vi "Write Data.vi"(8 "error in (no error)":errorcluster, 10 "Data":sgl, 11 "Single in":refnum<class "Single.lvclass">) -> (0 "error out":errorcluster, 3 "Single out":refnum<class "Single.lvclass">)   [LabVIEW 2019, in "Base Data Class.lvlib" / "Single.lvclass"]
uses:
  Single.lvclass
  Single.lvclass/Single.ctl
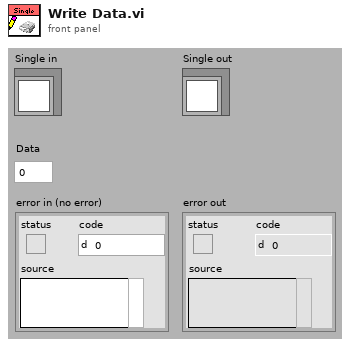
[diagram p1: front panel]
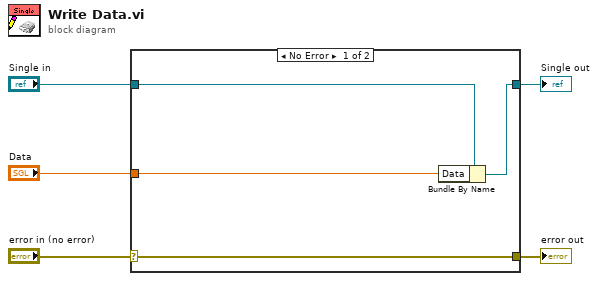
[diagram p0: block diagram]
diagram:
  n1 = case shown="No Error" "error in (no error)" {
    selector: "error in (no error)" -> [w9 w10]
    tunnel: [w9 w10] -> w4
    tunnel: [w7 w11] -> w2
    tunnel: "Single in" -> [w8 w11]
    tunnel: "Data" -> [w6 _]
    frame No Error {
      n2 = Bundle By Name(cluster=w8, "Data"=w6) -> (w7:refnum<class "Single.lvclass">)
    }
    frame Error {
    }
  }
  "error out" <- w4
  "Single out" <- w2
